vi "Agilent SNA Set Learn String.vi"(6 "Set SWP Learn String? (T)":bool=TRUE, 7 "Agilent SNA & SWP":T2, 8 "error in (no error)":errorcluster, 9 "SWP Learn String":string, 10 "SNA Learn String":string, 11 "VISA Resource Names":T1) -> (0 "error out":errorcluster {"code" format="%.0x"}, 3 "dup VISA Resource Names":T1)   [LabVIEW 2011]
uses:
  TypeDefs/Agilent SNA Instrument Info.ctl
  TypeDefs/Agilent SNA VISA.ctl
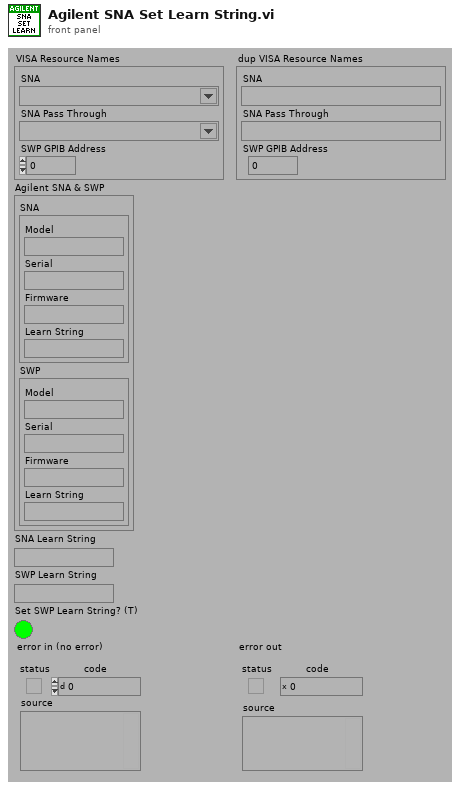
[diagram p1: front panel]
types:
  T1 = typedef "Agilent SNA VISA.ctl" = cluster{"SNA":refnum<visa-resource-name>, "SNA Pass Through":refnum<visa-resource-name>, "SWP GPIB Address":i32}
  T2 = typedef "Agilent SNA Instrument Info.ctl" = cluster{"SNA":cluster{"Model":string, "Serial":string, "Firmware":string, "Learn String":string}, "SWP":cluster{"Model":string, "Serial":string, "Firmware":string, "Learn String":string}}
  T3 = typedef "Agilent SNA Model.ctl" = enum16{"Not Supported", "8757X"}
  T4 = typedef "Agilent SNA SWP Model.ctl" = enum16{"Not Supported", "836XXX", "8375XX", "E82X7D"}
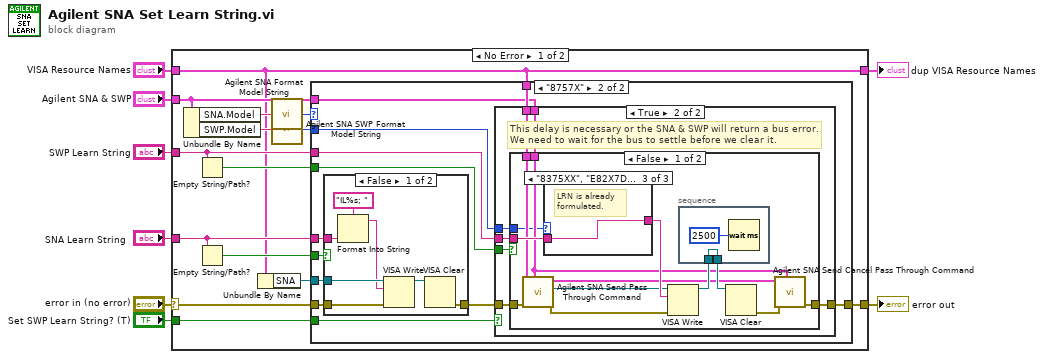
[diagram p0: block diagram]
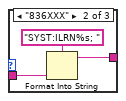
[diagram p5: hidden frame]
diagram:
  n1 = case shown="No Error" "error in (no error)" {
    selector: "error in (no error)" -> [w10 w73]
    tunnel: [w22 w73] -> w8
    tunnel: "SNA Learn String" -> [w20 _]
    tunnel: "SWP Learn String" -> [w16 _]
    tunnel: "VISA Resource Names" -> [w11 w72]
    tunnel: "Agilent SNA & SWP" -> [w14 _]
    tunnel: [w11 w72] -> w3
    tunnel: "Set SWP Learn String? (T)" -> [w9 _]
    frame No Error {
      n2 = Unbundle By Name(w14) -> ("SNA.Model"=w18:string, "SWP.Model"=w13:string)
      n3 = Empty String/Path?(string/path=w16) -> (empty?=w15:bool)
      n4 = Empty String/Path?(string/path=w20) -> (empty?=w21:bool)
      n5 = Unbundle By Name(w11) -> ("SNA"=w17:refnum<visa-resource-name>)
      n6 = call "Agilent SNA Format Model String.vi"("Model String"=w18) -> ("Model"=w19:T3)
      n7 = call "Agilent SNA SWP Format Model String.vi"("Model String"=w13) -> ("Model"=w12:T4)
      n8 = case shown="\"8757X\"" w19 {
        tunnel: [w23 w28] -> w22
        tunnel: w10 -> [w23 w35]
        tunnel: w21 -> [_ w34]
        tunnel: w20 -> [_ w33]
        tunnel: w17 -> [_ w32]
        tunnel: w16 -> [_ w31]
        tunnel: w15 -> [_ w30]
        tunnel: w11 -> [_ w27]
        tunnel: w14 -> [_ w26]
        tunnel: w12 -> [_ w25]
        tunnel: w9 -> [_ w24]
        frame "Not Supported" {
        }
        frame "8757X" {
          n9 = case shown="False" w34 {
            tunnel: [w68 w71] -> w29
            tunnel: w35 -> [w70 w71]
            tunnel: w33 -> [w67 _]
            tunnel: w32 -> [w69 _]
            frame False {
              n10 = Format Into String(format string="IL%s; ", w67) -> (resulting string=w65:string)  [unwired: 2 in, 1 out]
              n11 = VISA Write(VISA resource name=w69, write buffer=w65, error in (no error)=w70) -> (VISA resource name out=w64:refnum<visa-resource-name>)  [unwired: 2 out]
              n12 = VISA Clear(VISA resource name=w64) -> (error out=w68:errorcluster)  [unwired: 1 in, 1 out]
            }
            frame True {
            }
          }
          n13 = case shown="True" w24 {
            tunnel: w31 -> [_ w43]
            tunnel: w30 -> [_ w42]
            tunnel: w29 -> [w36 w41]
            tunnel: [w36 w40] -> w28
            tunnel: w27 -> [_ w39]
            tunnel: w26 -> [_ w38]
            tunnel: w25 -> [_ w37]
            frame False {
            }
            frame True {
              # "This delay is necessary or the SNA & SWP will return a bus error.\nWe need to wait for the bus to settle before we clear it."
              n14 = case shown="False" w42 {
                tunnel: [w48 w63] -> w40
                tunnel: w41 -> [w52 w63]
                tunnel: w43 -> [w54 _]
                tunnel: w39 -> [w50 _]
                tunnel: w38 -> [w46 _]
                tunnel: w37 -> [w44 _]
                frame False {
                  n15 = call "Agilent SNA Send Pass Through Command.vi"("Agilent SNA & SWP"=w46, "error in (no error)"=w52, "VISA Resource Names"=w50) -> ("error out"=w51:errorcluster, "SNA Pass Through"=w45:refnum<visa-resource-name>, "dup VISA Resource Names"=w47:T1)  [unwired: 1 in, 5 out]
                  n16 = case shown="\"8375XX\", \"E82X7D\"" w44 {
                    tunnel: w54 -> [_ w59 w60]
                    tunnel: [_ w57 w60] -> w53
                    frame "Not Supported" {
                    }
                    frame "836XXX" {
                      n17 = Format Into String(format string="SYST:ILRN%s; ", w59) -> (resulting string=w57:string)  [unwired: 2 in, 1 out]
                    }
                    frame "8375XX", "E82X7D" {
                      # "LRN is already\nformulated."
                    }
                  }
                  n18 = VISA Write(VISA resource name=w45, write buffer=w53, error in (no error)=w51) -> (VISA resource name out=w56:refnum<visa-resource-name>)  [unwired: 2 out]
                  n19 = stacked-sequence {
                    tunnel: w56 -> [w61]
                    tunnel: [w61] -> w55
                    frame #0 {
                      n20 = Wait (ms)(milliseconds to wait=u32 2500) -> ()  [unwired: 1 out]
                    }
                  }
                  n21 = VISA Clear(VISA resource name=w55) -> (error out=w49:errorcluster)  [unwired: 1 in, 1 out]
                  n22 = call "Agilent SNA Send Cancel Pass Through Command.vi"("Agilent SNA & SWP"=w46, "error in (no error)"=w49, "VISA Resource Names"=w47) -> ("error out"=w48:errorcluster)  [unwired: 1 in, 7 out]
                }
                frame True {
                }
              }
            }
          }
        }
      }
    }
    frame Error {
    }
  }
  "error out" <- w8
  "dup VISA Resource Names" <- w3
